vi "Stop Measurements.vi"(8 "error in (no error)":errorcluster, 11 "Pulse Controller in":refnum<class "Pulse Controller.lvclass">) -> (0 "error out":errorcluster, 3 "Pulse Controller out":refnum<class "Pulse Controller.lvclass">)   [LabVIEW 2015, in "Pulse Controller.lvclass"]
uses:
  Pulse Controller.lvclass
  Results/File Path Result/File Path Result.lvclass
  Measure Object/Measure Object.lvclass/Measure Object.ctl
  Results/Acquired Result/Acquired Result.lvclass/Acquired Result.ctl
  Plots/Plot types.ctl
  Measure Object Messages/Self-Addressed Msg/Self-addressed Msg.lvclass/Self-addressed Msg.ctl
  Measure_extentions/Monitor-Pulse Messages/Write Pulse File Msg/Write Pulse File Msg.lvclass/Write Pulse File Msg.ctl
  <vilib>/ActorFramework/Message Enqueuer/Message Enqueuer.lvclass/Message Enqueuer.ctl
  Measure Controller Messages/Open Waveform File Plot Msg/Open Waveform File Plot Msg.lvclass/Open Waveform File Plot Msg.ctl
  Measure Object Messages/Self-Addressed Msg/Read Return Enqueuer.vi
  Measure Object/Read tdms stream.vi
  Measure Object/Read Name.vi
  Results/Acquired Result/Write Sender.vi
  Measure Object/Read Reply to.vi
  <vilib>/ActorFramework/Message Enqueuer/Enqueue.vi
  Read Pulse Controller Configuration.vi
  <vilib>/ActorFramework/Message Priority Queue/Priority Enqueue.vi
  Measure Object Messages/Result Reply Msg/Result Reply Msg.lvclass
  <vilib>/ActorFramework/Message Enqueuer/Message Enqueuer.lvclass
  Measure_extentions/Monitor-Pulse Messages/Write Pulse File Msg/Write Pulse File Msg.lvclass
  Measure Controller Messages/Open Waveform File Plot Msg/Open Waveform File Plot Msg.lvclass
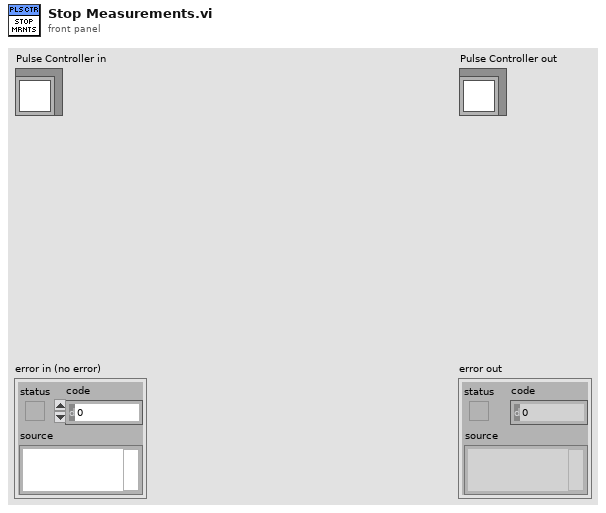
[diagram p1: front panel]
types:
  T1 = typedef "Pulse Controller Configuration.ctl" = cluster{"Pre-trigger duration":dbl, "Post-trigger duration":dbl, "Open plot after pulse":bool}
  T2 = typedef "Plot types.ctl" = enum16{"Waveform Plot", "XY Plot"}
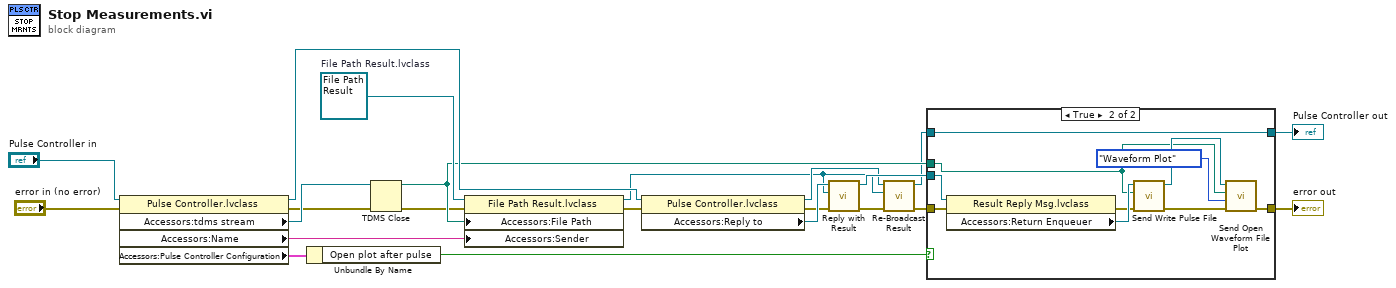
[diagram p0: block diagram]
diagram:
  w13 = refnum<class "File Path Result.lvclass"> refnum  # File Path Result.lvclass
  n1 = property class="Pulse Controller.lvclass"(reference="Pulse Controller in", error in="error in (no error)") -> (reference out=w14:refnum<class "Pulse Controller.lvclass">, error out=w19:errorcluster, "Accessors:tdms stream"=w21:refnum<k34>, "Accessors:Name"=w6:string, "Accessors:Pulse Controller Configuration"=w16:T1)
  n2 = Unbundle By Name(w16) -> ("Open plot after pulse"=w15:bool)
  n3 = TDMS Close(8:w19, 11:w21) -> (0:w11:errorcluster, 3:w12:path)
  n4 = property class="File Path Result.lvclass"(reference=w13, error in=w11, "Accessors:File Path"=w12, "Accessors:Sender"=w6) -> (reference out=w1:refnum<class "File Path Result.lvclass">, error out=w10:errorcluster)
  n5 = property class="Pulse Controller.lvclass"(reference=w14, error in=w10) -> (reference out=w5:refnum<class "Pulse Controller.lvclass">, error out=w8:errorcluster, "Accessors:Reply to"=w9:refnum<class "Result Reply Msg.lvclass">)
  n6 = call-dynamic "Reply with Result.vi"("error in (no error)"=w8, "Result"=w1, "Result Reply Msg in"=w9) -> ("error out"=w3:errorcluster, "Result Reply Msg out"=w7:refnum<class "Result Reply Msg.lvclass">)  [unwired: 7 in]
  n7 = call-dynamic "Re-Broadcast Result.vi"("error in (no error)"=w3, "Acquired Result.lvclass"=w1, "Measure Object in"=w5) -> ("error out"=w2:errorcluster, "Measure Object out"=w4:refnum<class "Pulse Controller.lvclass">)  [unwired: 7 in]
  n8 = case shown="True" w15 {
    tunnel: w4 -> [w24 w34]
    tunnel: [w24 w34] -> w18
    tunnel: w12 -> [_ w26]
    tunnel: w2 -> [w23 w33]
    tunnel: [w23 w32] -> w17
    tunnel: w7 -> [_ w31]
    frame False {
    }
    frame True {
      n9 = property class="Result Reply Msg.lvclass"(reference=w31, error in=w33) -> (error out=w27:errorcluster, "Accessors:Return Enqueuer"=w30:refnum<class "Message Enqueuer.lvclass">)  [unwired: 1 out]
      n10 = call "Send Write Pulse File.vi"("error in (no error)"=w27, "Pulse File"=w26, "Message Enqueuer"=w30) -> ("error out"=w28:errorcluster, "Message Enqueuer out"=w29:refnum<class "Message Enqueuer.lvclass">)  [unwired: 7 in]
      n11 = call "Send Open Waveform File Plot.vi"("error in (no error)"=w28, "Plot type"=Plot_types."Waveform Plot", "File Path Control"=w26, "Message Enqueuer"=w29) -> ("error out"=w32:errorcluster)  [unwired: 6 in, 1 out]
    }
  }
  "error out" <- w17
  "Pulse Controller out" <- w18
